vi "Get All Contacts.vi"(8 "error in (no error)":errorcluster) -> (0 "error out":errorcluster, 2 "Cursor List":T4, 3 "All Lines out":T1)   [LabVIEW 2014, in "Map Data.lvlib"]
doc: "Retrieves an array of all contacts in the address book data store."
uses:
  Map Data.lvlib
  CursorList.ctl
  All-Lines.ctl
  LineCluster.ctl
  LineConnection.ctl
  MapCommand.ctl
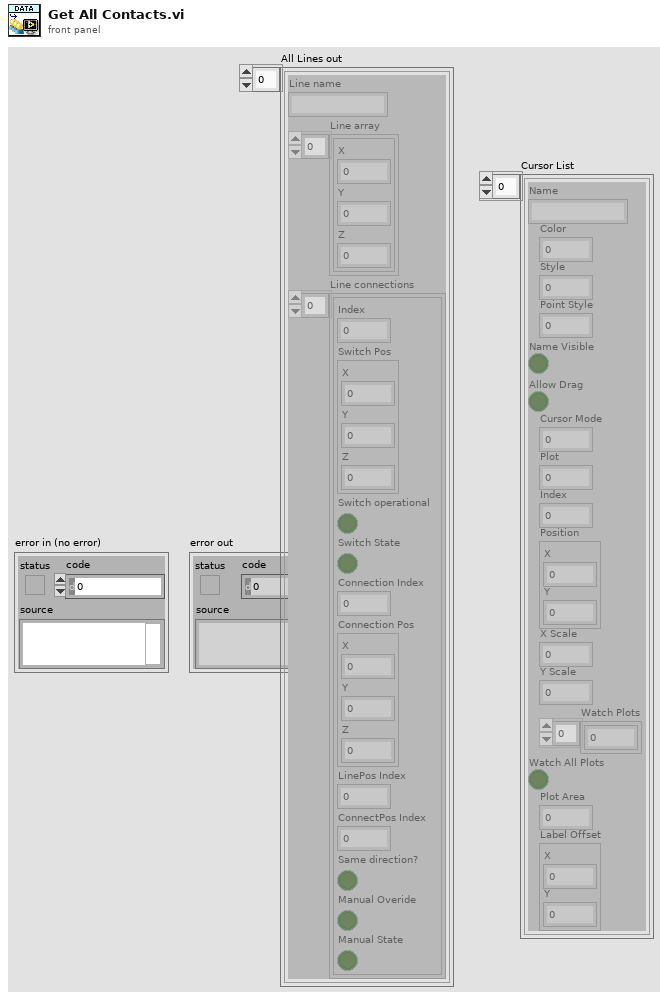
[diagram p1: front panel]
types:
  T1 = typedef "Map Data.lvlib/All-Lines.ctl" = T2[]
  T2 = typedef "Map Data.lvlib/LineCluster.ctl" = cluster{"Line name":string, "Line array":cluster{"X":dbl, "Y":dbl, "Z":dbl}[], "Line connections":T3[]}
  T3 = typedef "Map Data.lvlib/LineConnection.ctl" = cluster{"Index":i32, "Switch Pos":cluster{"X":dbl, "Y":dbl, "Z":dbl}, "Switch operational":bool, "Switch State":bool, "Connection Index":i32, "Connection Pos":cluster{"X":dbl, "Y":dbl, "Z":dbl}, "LinePos Index":i32, "ConnectPos Index":i32, "Same direction?":bool, "Manual Overide":bool, "Manual State":bool}
  T4 = typedef "Map Data.lvlib/CursorList.ctl" = cluster{"Name":string, "Color":u32, "Style":u8, "Point Style":u8, "Name Visible":bool, "Allow Drag":bool, "Cursor Mode":u32, "Plot":i32, "Index":i32, "Position":cluster{"X":dbl, "Y":dbl}, "X Scale":u32, "Y Scale":u32, "Watch Plots":i32[], "Watch All Plots":bool, "Plot Area":i32, "Label Offset":cluster{"X":dbl, "Y":dbl}}[]
  T5 = typedef "Map Data.lvlib/MapCommand.ctl" = enum16{"Load", "Update Cursor", "Save", "Get All Data", "Get Single Data", "Set Single Data", "Delete All", "Remove Single Data", "Set Favorite Status", "Is Data Modified", "Import Data"}
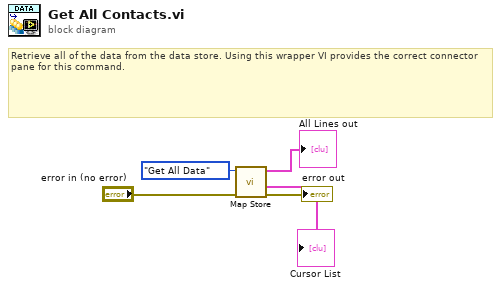
[diagram p0: block diagram]
diagram:
  # "Retrieve all of the data from the data store. Using this wrapper VI provides the correct connector pane for this command."
  n1 = call "Map Store.vi"("error in (no error)"="error in (no error)", "Command"=MapCommand."Get All Data") -> ("error out"=→"error out":errorcluster, "Cursor List"=→"Cursor List":T4, "All Lines out"=→"All Lines out":T1)  [unwired: 6 in, 1 out]
